vi "Test Class 1.vi"(9 "Boolean":bool, 10 "Numeric 2":dbl, 11 "Numeric":dbl) -> (3 "Test Class 1 out":refnum<class "Test Class 1.lvclass">)   [LabVIEW 2024, in "Test Class 1.lvclass"]
uses:
  Test Class 1.lvclass
  Test Class 1.lvclass/Test Class 1.ctl
panel:
  in  "Test Class 1.lvclass":refnum<class "Test Class 1.lvclass">
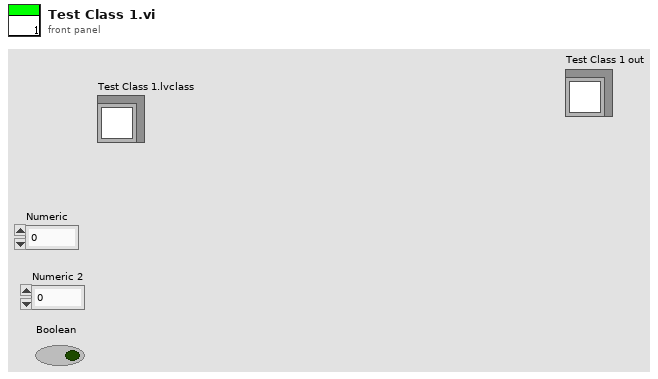
[diagram p1: front panel]
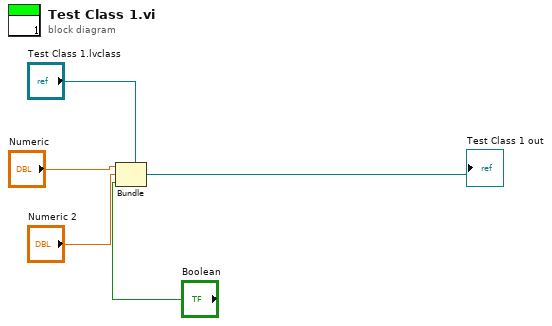
[diagram p0: block diagram]
diagram:
  n1 = Bundle(cluster="Test Class 1.lvclass", "Numeric", "Numeric 2", "Boolean") -> (→"Test Class 1 out":refnum<class "Test Class 1.lvclass">)
